vi "Write Config File.vi"(8 "Error In":errorcluster, 11 "UI Data in":T1={"SR Display List"=[], "Filter Cluster"={"Show Resolved"=TRUE, "Show Potentially Resolved"=TRUE, "Show Passoffs"=TRUE, "Show In Collab"=TRUE}, "Exit"=refnum, "Main VI"=refnum, "Sorting"=enum."SR Status", "Message"=refnum, "Legend"=refnum, "Sorting Reference"=refnum, "SR Display List Reference"=refnum, "Filter Cluster Reference"=refnum} {"SR Display List"."Creation Date" format="%<%x>T"; "SR Display List"."Last Updated" format="%<%x>T"}) -> (0 "Error Out":errorcluster, 3 "UI Data out":T1={"SR Display List"=[], "Filter Cluster"={"Show Resolved"=TRUE, "Show Potentially Resolved"=TRUE, "Show Passoffs"=TRUE, "Show In Collab"=TRUE}, "Exit"=refnum, "Main VI"=refnum, "Sorting"=enum."SR Status", "Message"=refnum, "Legend"=refnum, "Sorting Reference"=refnum, "SR Display List Reference"=refnum, "Filter Cluster Reference"=refnum} {"SR Display List"."Creation Date" format="%<%x>T"; "SR Display List"."Last Updated" format="%<%x>T"})   [LabVIEW 2018]
uses:
  Type Defs/UI Loop Data.ctl
  Type Defs/SR Cluster.ctl
  Type Defs/SR Status.ctl
  Type Defs/Filter Cluster.ctl
  Type Defs/Sorting Methods.ctl
  Type Defs/SR Display List Reference.ctl
  <vilib>/Utility/config.llb/Write Key (String).vi
  <vilib>/Utility/config.llb/Write Key (U32).vi
  <vilib>/Utility/config.llb/NI_LVConfig.lvlib
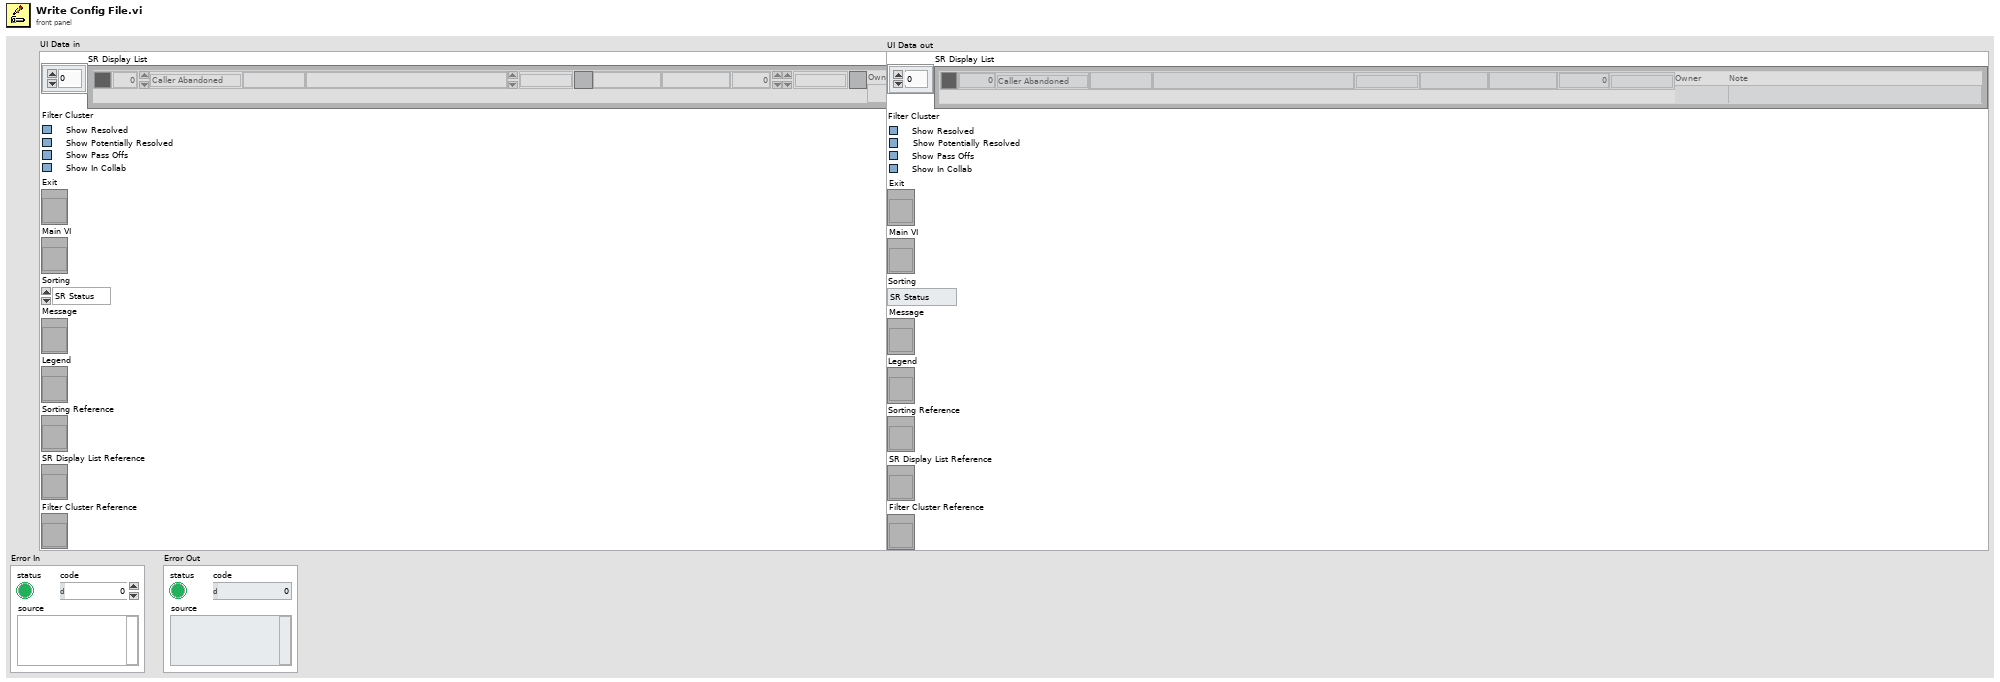
[diagram p1: front panel]
types:
  T1 = typedef "UI Loop Data.ctl" = cluster{"SR Display List":T2[], "Filter Cluster":T4, "Exit":refnum<vi>, "Main VI":refnum<vi>, "Sorting":T5, "Message":refnum<vi>, "Legend":refnum<vi>, "Sorting Reference":refnum<vi>, "SR Display List Reference":T6, "Filter Cluster Reference":refnum<vi>}
  T2 = typedef "SR Cluster.ctl" = cluster{"Color":u32, "SR Number":i32, "SR Status":T3, "Name":string, "Summary":string, "Last Updated":timestamp, "SR Type":string, "Service Level":string, "Days Open":dbl, "Creation Date":timestamp, "Owner":string, "Note":string}
  T3 = typedef "SR Status.ctl" = enum16{"Caller Abandoned", "Created in Error", "Expired", "Forum Resolved AE", "Forum Resolved Customer", "IN WORK", "IN WORK Collab with AES", "IN WORK Collab with PSE", "IN WORK Collab with SE", "IN WORK Customer Added Note", "IN WORK Escalation", "IN WORK Wait on Customer", "Open", "Potentially Resolved", "Presumed Resolved", "RMA Approved for Return", "RMA Closed", "RMA Closed - DOA", "RMA In Progress", "RMA Open", "RMA Waiting on Customer", "Resolved", "Passed Off"}
  T4 = typedef "Filter Cluster.ctl" = cluster{"Show Resolved":bool, "Show Potentially Resolved":bool, "Show Passoffs":bool, "Show In Collab":bool}
  T5 = typedef "Sorting Methods.ctl" = enum16{"SR Status", "Most Recent", "SR Type", "SR Number", "Days Open", "Urgency"}
  T6 = typedef "SR Display List Reference.ctl" = refnum<vi>
  T7 = typedef "NI_LVConfig.lvlib/Config Data RefNum.ctl" = refnum<k1>
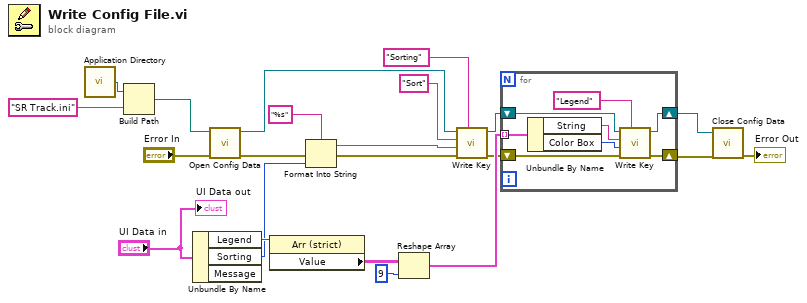
[diagram p0: block diagram]
diagram:
  n1 = call <vilib>:"Application Directory.vi"() -> ("Application Directory"=w20:path)
  n2 = Build Path(base path=w20, name or relative path="SR Track.ini") -> (appended path=w18:path)
  n3 = Unbundle By Name("UI Data in") -> ("Legend"=w21:refnum<vi>, "Sorting"=w17:T5)  [unwired: 1 out]
  n4 = call <vilib>:"Open Config Data.vi"("error in (no error)"="Error In", "configuration file path"=w18) -> ("error out"=w16:errorcluster, "refnum"=w13:T7)  [unwired: 7 in, 1 out]
  n5 = property class="Arr (strict)"(reference=w21) -> ("Value"=w8:cluster{"Color Box":u32, "String":string}[][])  [unwired: 1 in, 2 out]
  n6 = Format Into String(format string="%s", error in=w16, w17) -> (resulting string=w11:string, error out=w9:errorcluster)  [unwired: 1 in]
  n7 = Reshape Array(w8, 9 ("dimension size")) -> (w6:cluster{"Color Box":u32, "String":string}[])
  n8 = call-poly <vilib>:"Write Key.vi"("section"="Sorting", "error in (no error)"=w9, "value"=w11, "key"="Sort", "refnum"=w13) -> ("error out"=w4:errorcluster, "refnum out"=w5:T7)  [unwired: 4 in, 1 out]
  n9 = for {
    tunnel: w6 -> [w30] mode=indexing
    shift-right: [w25] -> w1
    shift-left: w4 -> [w26]
    shift-right: [w27] -> w2
    shift-left: w5 -> [w28]
    n10 = Unbundle By Name(w30) -> ("String"=w23:string, "Color Box"=w24:u32)
    n11 = call-poly <vilib>:"Write Key.vi"("section"="Legend", "error in (no error)"=w26, "value"=w24, "key"=w23, "refnum"=w28) -> ("error out"=w25:errorcluster, "refnum out"=w27:T7)  [unwired: 4 in, 1 out]
  }
  n12 = call <vilib>:"Close Config Data.vi"("error in (no error)"=w1, "refnum"=w2) -> ("error out"=→"Error Out":errorcluster)  [unwired: 8 in, 1 out]
  "UI Data out" <- "UI Data in"
